vi "workspace.clear.vi"(8 "error in":errorcluster, 11 "Nominal Client in":refnum<class "Nominal Client.lvclass">) -> (0 "error out":errorcluster, 3 "Nominal Client out":refnum<class "Nominal Client.lvclass">)   [LabVIEW 2020, in "Nominal Client.lvclass"]
doc: "If cleared or not provided, the client will use the default workspace for the user’s organization, if the default workspace for the organization is configured."
uses:
  Nominal Client.lvclass
  nominal types/workspace/workspace.lvclass
  Nominal Client.lvclass/Nominal Client.ctl
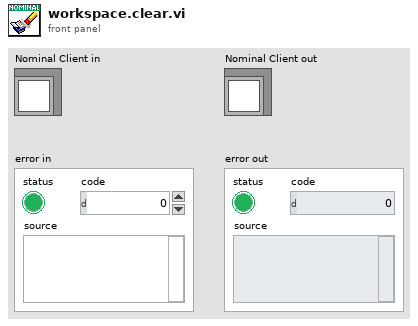
[diagram p1: front panel]
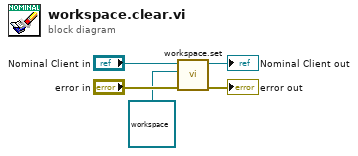
[diagram p0: block diagram]
diagram:
  n1 = call "workspace.set.vi"("error in"="error in", "workspace"=refnum<class "workspace.lvclass"> refnum, "Nominal Client in"="Nominal Client in") -> ("error out"=→"error out":errorcluster, "Nominal Client out"=→"Nominal Client out":refnum<class "Nominal Client.lvclass">)  [unwired: 7 in]
